vi "Uint32Array Create (Dimensions).vi"(8 "error in (no error)":errorcluster, 10 "Array dimensions":i32[](array[numeric]), 11 "U32 array in":u32[](array[numeric])) -> (0 "error out":errorcluster, 3 "Uint32Array DVR out":refnum<data-value>)   [LabVIEW 2012, in "MDSplus.lvlib"]
uses:
  <vilib>/MDSplus/Library/MDSplus.lvlib
  <vilib>/MDSplus/Classes/Data_Class/Array_Class/Uint32Array_Class/Uint32Array.lvclass
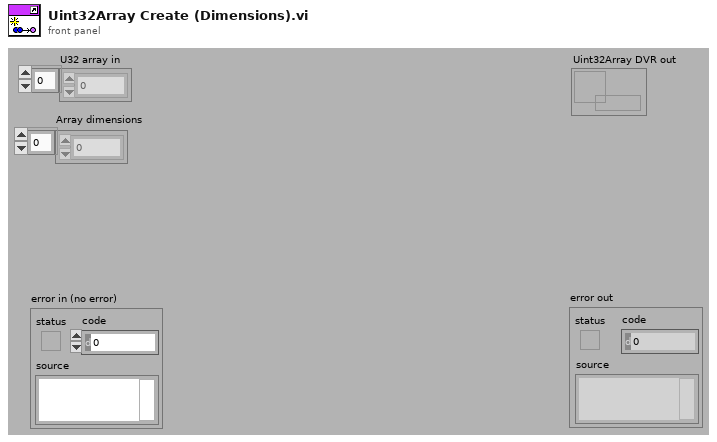
[diagram p1: front panel]
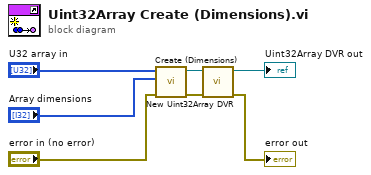
[diagram p0: block diagram]
diagram:
  n1 = call <vilib>:"Create (Dimensions).vi"("error in (no error)"="error in (no error)", "Dimensions"="Array dimensions", "U32 array in"="U32 array in") -> ("error out"=w4:errorcluster, "Uint32Array out"=w5:refnum<class "Uint32Array.lvclass">)  [unwired: 7 in]
  n2 = call <vilib>:"New Uint32Array DVR.vi"("error in (no error)"=w4, "Uint32Array in"=w5) -> ("error out"=→"error out":errorcluster, "Uint32Array DVR out"=→"Uint32Array DVR out":refnum<data-value>)  [unwired: 8 in]
